vi "N9310A Sweep LF.vi"() -> ()   [LabVIEW 2018]
uses:
  <instrlib>/Agilent N9310/Agilent N9310.lvlib
panel:
  in  "VISA resource name of Agilent N9310A":refnum<visa-resource-name>
  in  "Wait between steps (s)":dbl format="%#_6p"
  out "Current step":dbl format="%^#_6e"
  out "Current frequency":dbl format="%#_6p"
  in  "Steps":dbl format="%^#_6e"
  in  "Amplitude (V)":dbl format="%#_6p"
  in  "End frequency (Hz)":dbl format="%#_6p"
  in  "Start frequency (Hz)":dbl format="%#_6p"
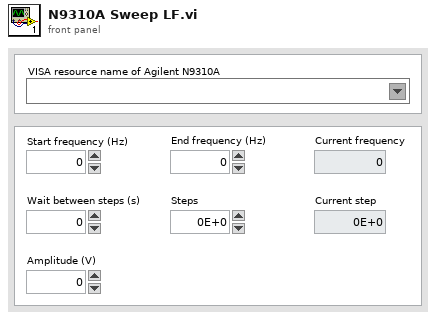
[diagram p1: front panel]
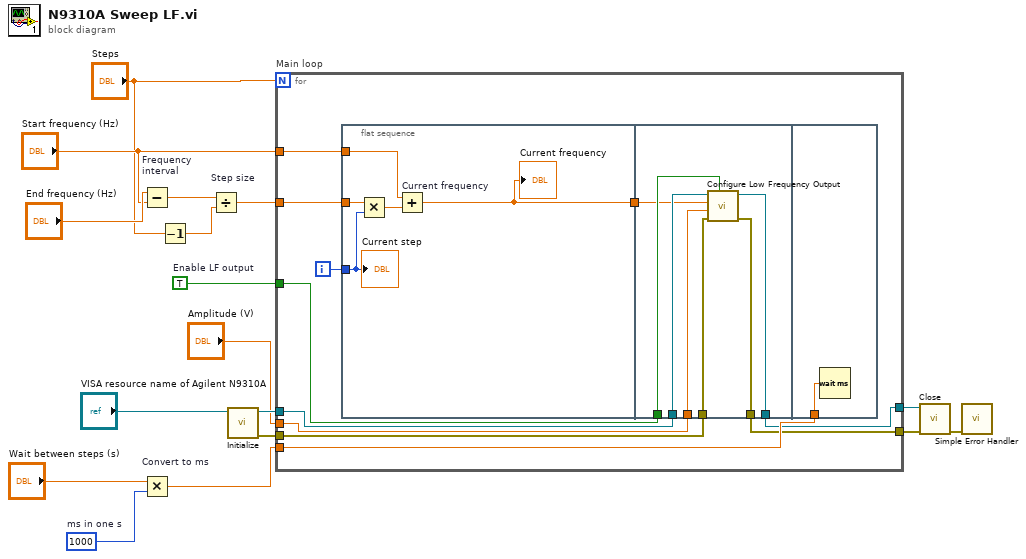
[diagram p0: block diagram]
diagram:
  w5 = TRUE  # Enable LF output
  w11 = 1000  # ms in one s
  n1 = Subtract "Frequency\ninterval"(x="End frequency (Hz)", y="Start frequency (Hz)") -> (x-y=w16:dbl)
  n2 = Multiply "Convert to ms"(x="Wait between steps (s)", y=w11) -> (x*y=w13:dbl)
  n3 = Decrement(x="Steps") -> (x-1=w9:dbl)
  n4 = Divide "Step size"(x=w16, y=w9) -> (x/y=w15:dbl)
  n5 = call <instrlib>:"Initialize.vi"("VISA resource name"="VISA resource name of Agilent N9310A") -> ("error out"=w6:errorcluster, "VISA resource name out"=w7:refnum<visa-resource-name>)  [unwired: 9 in]
  n6 = for "Main loop" {
    N: "Steps" -> [_]
    tunnel: w15 -> [w28]
    tunnel: "Start frequency (Hz)" -> [w27]
    tunnel: w13 -> [w26]
    tunnel: w7 -> [w25]
    tunnel: w6 -> [w24]
    tunnel: w5 -> [w23]
    tunnel: "Amplitude (V)" -> [w21]
    tunnel: [w20] -> w2
    tunnel: [w19] -> w1
    i -> [w18]
    n7 = flat-sequence {
      tunnel: w18 -> [w29]
      tunnel: w28 -> [w32]
      tunnel: w27 -> [w31]
      tunnel: [w30] -> w22
      tunnel: w25 -> [w40]
      tunnel: w24 -> [w39]
      tunnel: w23 -> [w38]
      tunnel: w22 -> [w37]
      tunnel: w21 -> [w36]
      tunnel: [w35] -> w20
      tunnel: [w34] -> w19
      tunnel: w26 -> [w41]
      frame #0 {
        n8 = Multiply(x=w32, y=w29) -> (x*y=w33:dbl)
        n9 = Add "Current frequency"(x=w31, y=w33) -> (x+y=w30:dbl)
        "Current frequency" <- w30
        "Current step" <- w29
      }
      frame #1 {
        n10 = call <instrlib>:"Configure Low Frequency Output.vi"("Enable LF Output (F:Disable)"=w38, "error in (no error)"=w39, "Amplitude (0.5 V)"=w36, "Frequency (1.0 kHz)"=w37, "VISA resource name"=w40) -> ("error out"=w34:errorcluster, "VISA resource name out"=w35:refnum<visa-resource-name>)  [unwired: 5 in]
      }
      frame #2 {
        n11 = Wait (ms)(milliseconds to wait=w41) -> ()  [unwired: 1 out]
      }
    }
  }
  n12 = call <instrlib>:"Close.vi"("error in (no error)"=w1, "VISA resource name"=w2) -> ("error out"=w3:errorcluster)  [unwired: 9 in]
  n13 = call <vilib>:"Simple Error Handler.vi"("error in (no error)"=w3) -> ()  [unwired: 4 in, 5 out]
